vi "availableIDs.vi"(8 "error in (no error)":errorcluster, 10 "NumberOfIDs":u32=1, 11 "Structure in":refnum<class "Structure.lvclass">) -> (0 "error out":errorcluster, 2 "IDs":u32[](array[numeric]), 3 "Structure out":refnum<class "Structure.lvclass">)   [LabVIEW 2009, in "Structure.lvclass"]
doc: "Searches the Node list for unique IDs to be assigned to nodes"
uses:
  Structure.lvclass
  Structure.lvclass/Structure.ctl
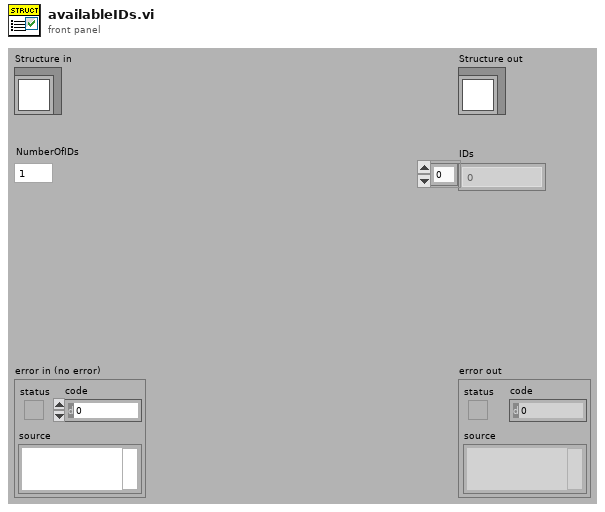
[diagram p1: front panel]
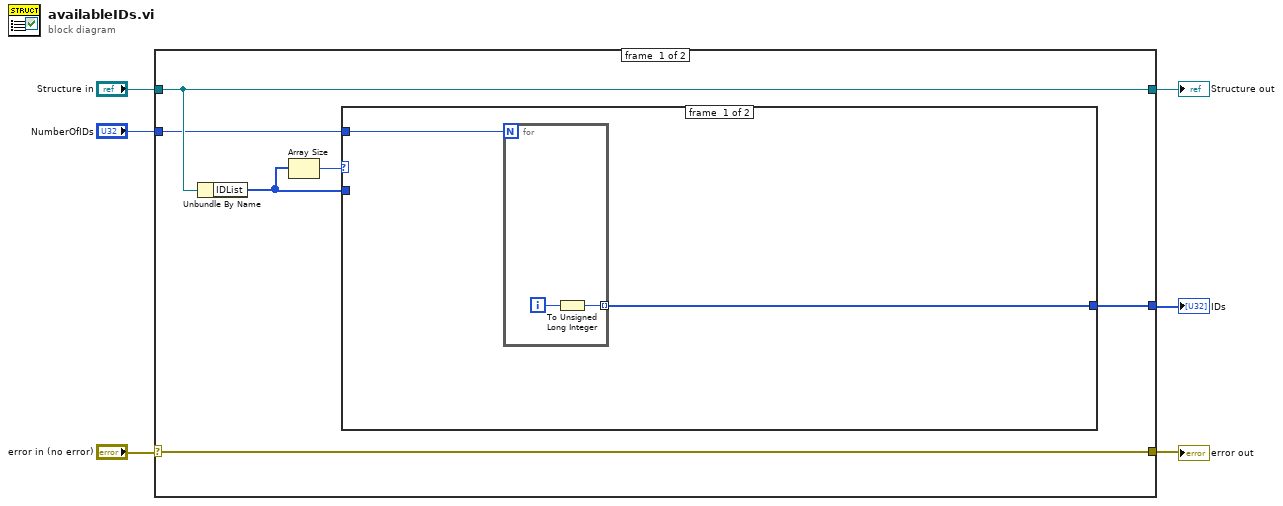
[diagram p0: block diagram]
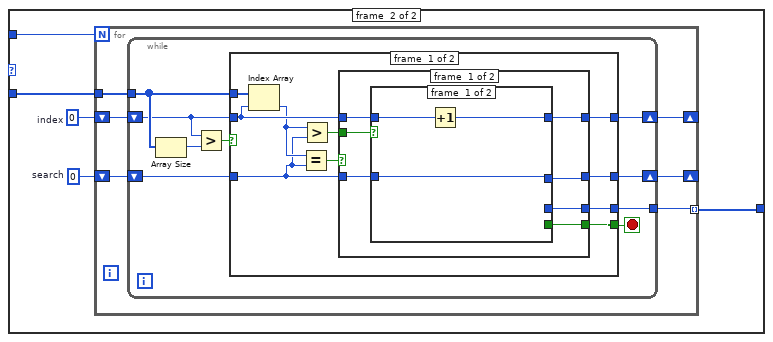
[diagram p2: hidden frame]
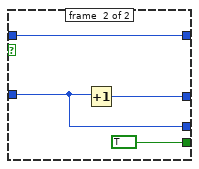
[diagram p3: hidden frame]
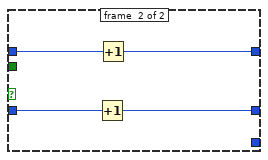
[diagram p4: hidden frame]
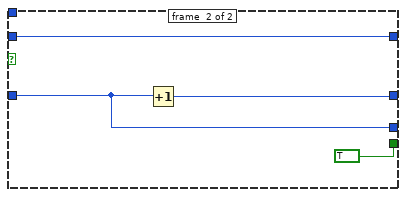
[diagram p5: hidden frame]
diagram:
  n1 = case shown="No Error" "error in (no error)" {
    selector: "error in (no error)" -> [w12 w70]
    tunnel: [w12 w70] -> w1
    tunnel: [w11 w69] -> w5
    tunnel: "Structure in" -> [w11 w69]
    tunnel: "NumberOfIDs" -> [w10 _]
    tunnel: [w9 _] -> w4
    frame #0 {
      n2 = Unbundle By Name(w11) -> ("IDList"=w7:u32[])
      n3 = Array Size(array=w7) -> (size(s)=w8:i32)
      n4 = case shown="Default" w8 {
        tunnel: w10 -> [w14 w21]
        tunnel: [w13 w20] -> w9
        tunnel: w7 -> [_ w17]
        frame #0 {
          n5 = for {
            N: w14 -> [_]
            tunnel: [w15] -> w13 mode=indexing
            i -> [w16]
            n6 = To Unsigned Long Integer(number=w16) -> (unsigned 32bit integer=w15:u32)
          }
        }
        frame #1 {
          w18 = u32 0  # search
          w19 = 0  # index
          n7 = for {
            N: w21 -> [_]
            shift-right: [w24] -> _
            shift-left: w19 -> [w26]
            shift-right: [w22] -> _
            shift-left: w18 -> [w25]
            tunnel: w17 -> [w27]
            tunnel: [w23] -> w20 mode=indexing
            n8 = while {
              tunnel: w27 -> [w30]
              shift-right: [w35] -> w22
              shift-left: w25 -> [w32]
              shift-right: [w34] -> w24
              shift-left: w26 -> [w28]
              tunnel: [w33] -> w23
              stop <- w36 stop-if-true
              n9 = Array Size(array=w30) -> (size(s)=w29:i32)
              n10 = Greater?(x=w28, y=w29) -> (0:w31:bool)
              n11 = case shown="False" w31 {
                tunnel: w28 -> [w45 w68]
                tunnel: [w44 TRUE] -> w36
                tunnel: [w43 w67] -> w35
                tunnel: [w42 w68] -> w34
                tunnel: w32 -> [w40 w66]
                tunnel: [w38 w66] -> w33
                tunnel: w30 -> [w37 _]
                frame #0 {
                  n12 = Index Array(array=w37, index=w45) -> (element=w41:u32)
                  n13 = Equal?(x=w41, y=w40) -> (x = y?=w46:bool)
                  n14 = Greater?(x=w41, y=w40) -> (0:w39:bool)
                  n15 = case shown="False" w46 {
                    tunnel: w45 -> [w52 w62]
                    tunnel: w40 -> [w50 w64]
                    tunnel: [w47 _] -> w44
                    tunnel: [w49 w63] -> w43
                    tunnel: [w51 w61] -> w42
                    tunnel: w39 -> [w53 _]
                    tunnel: [w48 _] -> w38
                    frame #0 {
                      n16 = case shown="False" w53 {
                        tunnel: w52 -> [w56 w60]
                        tunnel: [w54 w60] -> w51
                        tunnel: w50 -> [w55 w58]
                        tunnel: [w55 w59] -> w49
                        tunnel: [_ w58] -> w48
                        tunnel: [_ TRUE] -> w47
                        frame #0 {
                          n17 = Increment(x=w56) -> (x+1=w54:i32)
                        }
                        frame #1 {
                          n18 = Increment(x=w58) -> (x+1=w59:u32)
                        }
                      }
                    }
                    frame #1 {
                      n19 = Increment(x=w64) -> (x+1=w63:u32)
                      n20 = Increment(x=w62) -> (x+1=w61:i32)
                    }
                  }
                }
                frame #1 {
                  n21 = Increment(x=w66) -> (x+1=w67:u32)
                }
              }
            }
          }
        }
      }
    }
    frame #1 {
    }
  }
  "error out" <- w1
  "Structure out" <- w5
  "IDs" <- w4
